vi "Stop Waveform Generation.vi"(8 "error in (no error)":errorcluster, 11 "Hw sync command Q":refnum<queue>) -> ()   [LabVIEW 2021, in "audio adc shared.lvlib"]
uses:
  controls/Sync Commands.ctl
  audio adc shared.lvlib
  controls/audio adc controls.lvlib
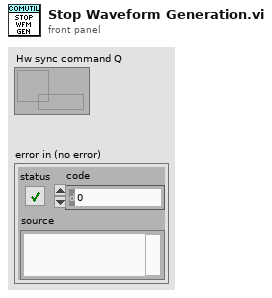
[diagram p1: front panel]
types:
  T1 = typedef "audio adc controls.lvlib/Sync Commands.ctl" = enum16{"NoAction", "GenerationStarted", "AcquisitionCompleted", "GenerationErrored"}
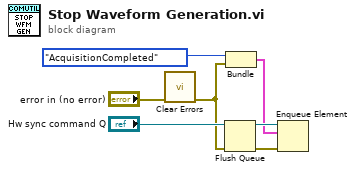
[diagram p0: block diagram]
diagram:
  n1 = call <vilib>:"Clear Errors.vi"("error in (no error)"="error in (no error)") -> ("error out"=w3:errorcluster)  [unwired: 5 in, 1 out]
  n2 = Flush Queue(queue="Hw sync command Q", error in (no error)=w3) -> (queue out=w2:refnum<queue>, error out=w4:errorcluster)  [unwired: 1 out]
  n3 = Bundle("Status"=Sync_Commands."AcquisitionCompleted", "error out"=w3) -> (w1:cluster{"Status":T1, "error out":errorcluster})  [unwired: 1 in]
  n4 = Enqueue Element(queue=w2, element=w1, error in (no error)=w4) -> ()  [unwired: 1 in, 3 out]
